vi "Write Class Name.vi"(10 "Class Name":string, 11 "Message Scripter in":refnum<class "Message Scripter.lvclass">) -> (3 "Message Scripter out":refnum<class "Message Scripter.lvclass">)   [LabVIEW 2020, in "Message Maker.lvlib" / "Message Scripter.lvclass"]
uses:
  Message Scripter.lvclass
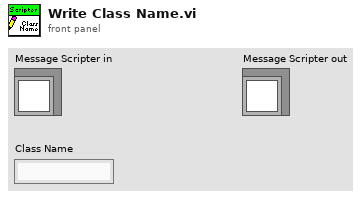
[diagram p1: front panel]
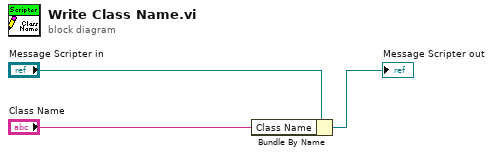
[diagram p0: block diagram]
diagram:
  n1 = Bundle By Name(cluster="Message Scripter in", "Class Name"="Class Name") -> (→"Message Scripter out":refnum<class "Message Scripter.lvclass">)
